vi "Test Stamp Grab and Replace.vi"() -> ()   [LabVIEW 2011]
uses:
  CameraTool Class/Type Definitions/Fiducial Acquisition Parameters.ctl
  Config Manager Class/Type Definitions/Fiducial Type.ctl
  WorkTable Class/Type Definitions/Worktable_Stamp.ctl
  Utils/Type Definitions/Position_Orientation.ctl
  Vec3d Class/Vec3d Class.lvclass
  Orient3d Class/Orient3d Class.lvclass
  Config Manager Class/Type Definitions/Stamp Type.ctl
  CameraTool Class/CameraTool Class.lvclass
  GrabberTool Class.lvclass
  Gantry Class/Gantry Class.lvclass
  Config Manager Class/Config Manager Class.lvclass
  WorkTable Class/WorkTable Class.lvclass
panel:
  out "error out":errorcluster
  in  "Position":string
  in  "Orientation":string
  in  "Config Folder":path=path "C:/Users/husker/Desktop/gantry/Config"
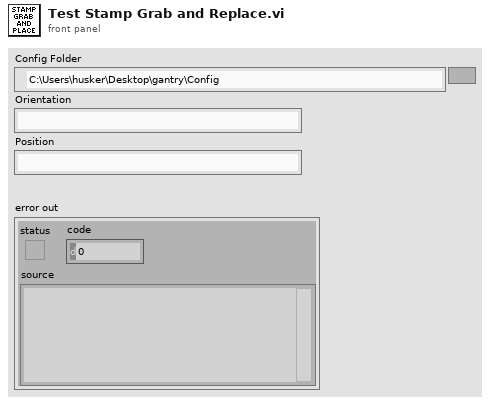
[diagram p1: front panel]
types:
  T1 = typedef "Position_Orientation.ctl" = cluster{"Center":refnum<class "Vec3d Class.lvclass">, "Orientation":refnum<class "Orient3d Class.lvclass">}
  T2 = typedef "Stamp Type.ctl" = enum16{"Stamp 1", "Stamp 2", "Stamp 3", "Stamp 4", "Stamp 5"}
  T3 = typedef "Worktable_Stamp.ctl" = cluster{"Stamp State":enum16{"Empty", "Populated", "Used"}, "Location/Orientation":T1, "Stamp Type":T2}
  T4 = typedef "Fiducial Type.ctl" = enum16{"HDI", "BBM"}
  T5 = typedef "Fiducial Acquisition Parameters.ctl" = cluster{"Selection Criteria":enum16{"Single", "Top", "Bottom"}, "Image Prefix":string, "Fiducial Type":T4}
  T6 = cluster{"Feature Coordinates":refnum<class "Vec3d Class.lvclass">, "Feature Name":string}[]
  T7 = typedef "Fiducial Image.ctl" = cluster{"Fiducial Image":T8, "Selected Fiducial":T10, "fiducial name":string}
  T8 = typedef "Physical Image.ctl" = cluster{"Image Position":refnum<class "Vec3d Class.lvclass">, "Image Reference":T9, "Field of View":cluster{"x(mm)":dbl, "y(mm)":dbl}}
  T9 = typedef "IMAQ Image.ctl" = refnum<image>
  T10 = typedef "Fiducial with Source.ctl" = cluster{"Fiducial Image Coordinate":refnum<class "Vec3d Class.lvclass">, "Fiducial Source":enum16{"Pattern Recognition", "User", "Error", "Default"}}
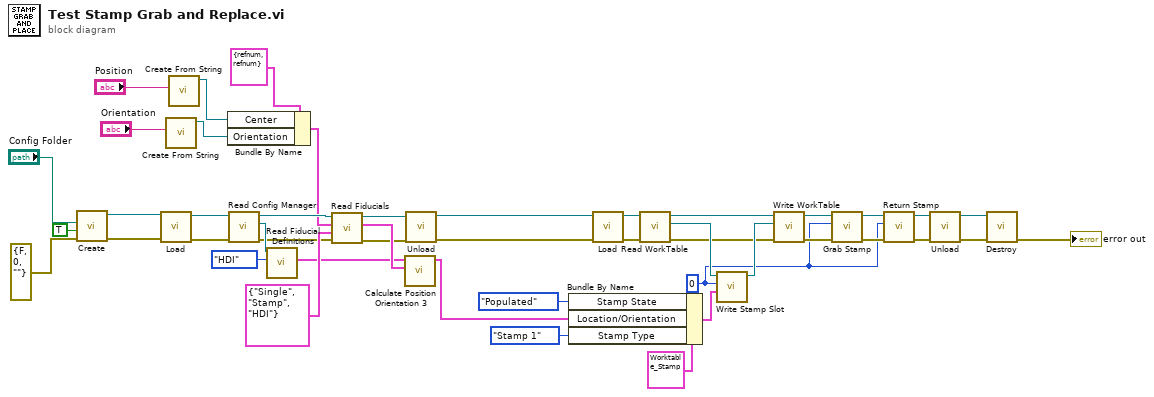
[diagram p0: block diagram]
diagram:
  w2 = 0 ("Stamp Slot")
  n1 = call "Create.vi"("error in"=errorcluster {"status"=FALSE, "code"=0, "source"=""}, "HOME?"=TRUE, "Config Folder"="Config Folder") -> ("error out"=w15:errorcluster, "Gantry out"=w44:refnum<class "Gantry Class.lvclass">)  [unwired: 7 in]
  n2 = call "Load.vi"("error in"=w15, "Gantry In"=w44) -> ("error out"=w13:errorcluster, "CameraTool out"=w39:refnum<class "CameraTool Class.lvclass">)  [unwired: 8 in]
  n3 = call "Create From String.vi"("Input String"="Orientation") -> ("Orient3d out"=w17:refnum<class "Orient3d Class.lvclass">)  [unwired: 9 in, 1 out]
  n4 = call "Create From String.vi"("Input String"="Position") -> ("Vec3d out"=w18:refnum<class "Vec3d Class.lvclass">)  [unwired: 9 in, 1 out]
  n5 = Bundle By Name(cluster=T1 {"Center"=refnum, "Orientation"=refnum} ("Location/Orientation in"), "Center"=w18, "Orientation"=w17) -> (w16:T1)
  n6 = call-dynamic "Read Config Manager.vi"("error in"=w13, "Gantry in"=w39) -> ("error out"=w12:errorcluster, "Config Manager"=w38:refnum<class "Config Manager Class.lvclass">, "Gantry out"=w37:refnum<class "CameraTool Class.lvclass">)  [unwired: 7 in]
  n7 = call "Read Fiducial Definitions.vi"("Fiducial Type"=Fiducial_Type."HDI", "Config Manager in"=w38) -> ("Feature Definitions"=w41:T6)  [unwired: 7 in, 2 out]
  n8 = call-dynamic "Read Fiducials.vi"("error in"=w12, "Fiducial Acquisition Parameters"=T5 {"Selection Criteria"=enum."Single", "Image Prefix"="Stamp", "Fiducial Type"=enum."HDI"}, "Location/Orientation in"=w16, "CameraTool in"=w37) -> ("error out"=w11:errorcluster, "Fiducials"=w42:T7[], "CameraTool out"=w36:refnum<class "CameraTool Class.lvclass">)  [unwired: 5 in]
  n9 = call "Calculate Position Orientation 3.vi"("Fiducials"=w42, "Feature Definitions"=w41) -> ("PositionOrientation"=w25:T1)  [unwired: 8 in, 1 out]
  n10 = call "Unload.vi"("error in"=w11, "CameraTool in"=w36) -> ("error out"=w10:errorcluster, "Gantry out"=w35:refnum<class "Gantry Class.lvclass">)  [unwired: 8 in]
  n11 = Bundle By Name(cluster=T3 {"Stamp State"=enum."Empty", "Location/Orientation"={"Center"=refnum, "Orientation"=refnum}, "Stamp Type"=enum."Stamp 1"} ("Stamp Slot"), "Stamp State"=enum16{"Empty", "Populated", "Used"}."Populated", "Location/Orientation"=w25, "Stamp Type"=Stamp_Type."Stamp 1") -> (w24:T3)
  n12 = call "Load.vi"("error in"=w10, "Gantry In"=w35) -> ("error out"=w9:errorcluster, "Grabber Tool out"=w29:refnum<class "GrabberTool Class.lvclass">)  [unwired: 8 in]
  n13 = call-dynamic "Read WorkTable.vi"("error in"=w9, "Gantry Class in"=w29) -> ("error out"=w8:errorcluster, "WorkTable Class.lvclass"=w28:refnum<class "WorkTable Class.lvclass">, "Gantry Class out"=w27:refnum<class "GrabberTool Class.lvclass">)  [unwired: 7 in]
  n14 = call "Write Stamp Slot.vi"(9:"Stamp Slot"=w24, 10:"Stamp Slot"=w2, "WorkTable Class in"=w28) -> ("WorkTable Class out"=w31:refnum<class "WorkTable Class.lvclass">)  [unwired: 7 in, 1 out]
  n15 = call-dynamic "Write WorkTable.vi"("error in (no error)"=w8, "WorkTable Class.lvclass"=w31, "Gantry Class in"=w27) -> ("error out"=w7:errorcluster, "Gantry Class out"=w30:refnum<class "GrabberTool Class.lvclass">)  [unwired: 7 in]
  n16 = call "Grab Stamp.vi"("error in"=w7, "Stamp Number"=w2, "GrabberTool in"=w30) -> ("error out"=w6:errorcluster, "GrabberTool out"=w34:refnum<class "GrabberTool Class.lvclass">)  [unwired: 7 in]
  n17 = call "Return Stamp.vi"("error in"=w6, "Slot Number"=w2, "GrabberTool in"=w34) -> ("error out"=w5:errorcluster, "GrabberTool out"=w33:refnum<class "GrabberTool Class.lvclass">)  [unwired: 7 in]
  n18 = call "Unload.vi"("error in"=w5, "GrabberTool in"=w33) -> ("error out"=w4:errorcluster, "Gantry out"=w32:refnum<class "Gantry Class.lvclass">)  [unwired: 8 in]
  n19 = call "Destroy.vi"("error in"=w4, "Gantry Class in"=w32) -> ("error out"=→"error out":errorcluster)  [unwired: 9 in]
